vi "Generate File Name.vi"(6 "Y":i32, 7 "X":i32, 8 "Z":i32, 9 "path":path=path "C:/Users/BOAS-USER/Documents/Data/0507/human", 10 "#C scan":i32, 11 "Channel":i32) -> (3 "appended path":path)   [LabVIEW 2018]
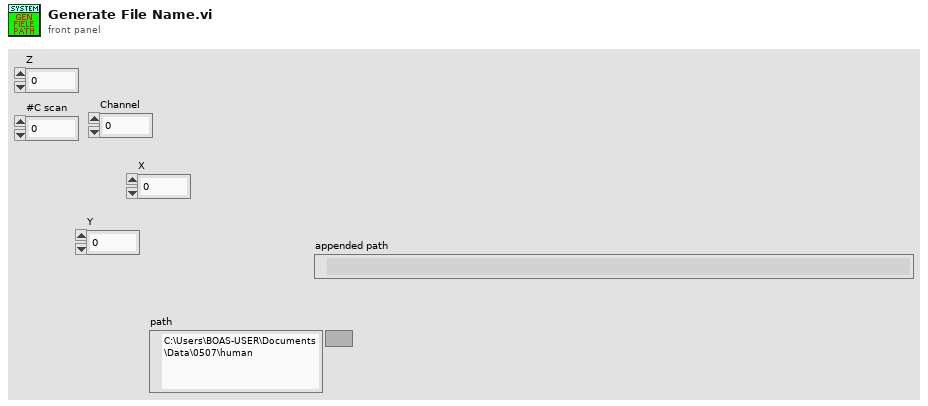
[diagram p1: front panel]
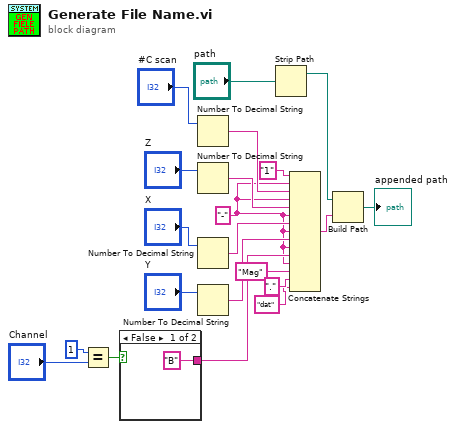
[diagram p0: block diagram]
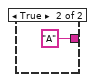
[diagram p2: hidden frame]
diagram:
  w4 = "-" ("string")
  n1 = Equal?(x=u32 1, y="Channel") -> (x = y?=w18:bool)
  n2 = case shown="False" w18 {
    tunnel: ["B" "A"] -> w7
    frame False {
    }
    frame True {
    }
  }
  n3 = Number To Decimal String(number="#C scan") -> (decimal integer string=w13:string)  [unwired: 1 in]
  n4 = Number To Decimal String(number="Z") -> (decimal integer string=w12:string)  [unwired: 1 in]
  n5 = Number To Decimal String(number="X") -> (decimal integer string=w10:string)  [unwired: 1 in]
  n6 = Number To Decimal String(number="Y") -> (decimal integer string=w8:string)  [unwired: 1 in]
  n7 = Strip Path(path="path") -> (stripped path=w15:path)  [unwired: 1 out]
  n8 = Concatenate Strings("1" ("string"), w4, w13, w4, w12, w4, w10, w4, w8, w4, w7, w4, "Mag" ("string"), "." ("string"), "dat" ("string")) -> (w5:string)
  n9 = Build Path(base path=w15, name or relative path=w5) -> (appended path=→"appended path":path)
